vi "CMN_processOneExt.vi"(8 "error in (no error)":errorcluster, 9 "starting line":u16, 10 "str in":string) -> (0 "error out":errorcluster, 2 "number of keywords found":i32, 3 "HdrInfo":string[][](table))   [LabVIEW 2016]
doc: "This VI reads the configuration file searching for the \"infofile\" keyword. Then, it goes and reads the specified file, which should be a template for the TCS info format"
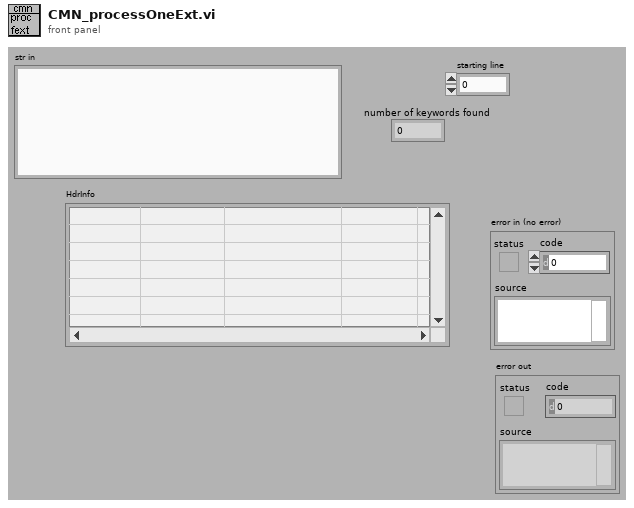
[diagram p1: front panel]
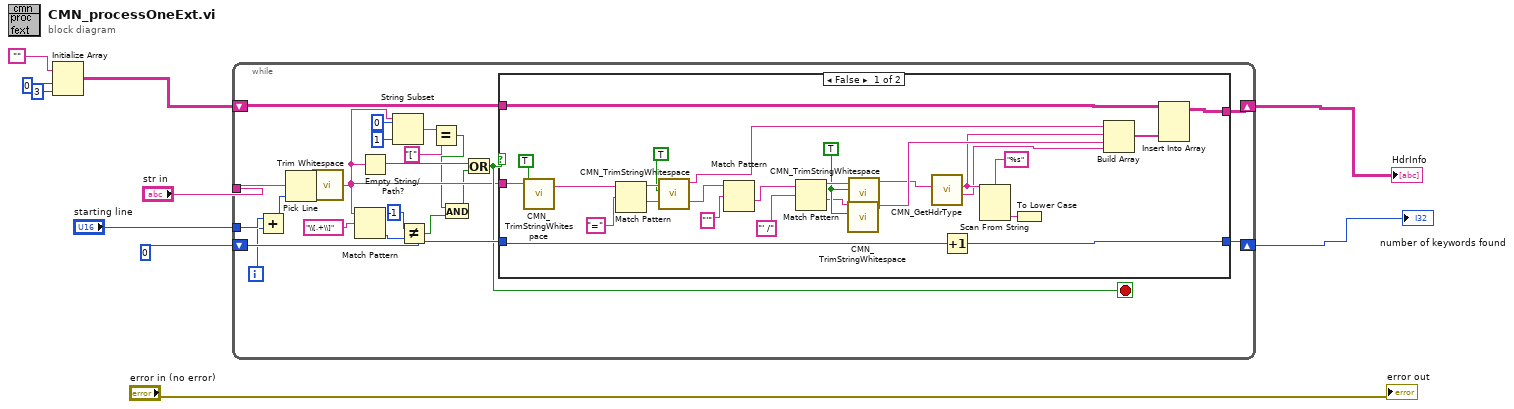
[diagram p0: block diagram]
diagram:
  n1 = Initialize Array("", 0, 3 ("dimension size")) -> (w6:string[][])
  n2 = while {
    shift-left: 0 -> [w25]
    shift-right: [w26] -> w8
    shift-left: w6 -> [w31]
    shift-right: [w30] -> w9
    tunnel: "str in" -> [w32]
    tunnel: "starting line" -> [w22]
    i -> [w21]
    stop <- w19 stop-if-true
    n3 = Add(x=w22, y=w21) -> (x+y=w20:i32)
    n4 = Pick Line(multi-line string=w32, line index=w20) -> (output string=w23:string)  [unwired: 1 out]
    n5 = call <vilib>:"Trim Whitespace.vi"("string"=w23) -> ("trimmed string"=w16:string)  [unwired: 1 in]
    n6 = Match Pattern(string=w16, regular expression="\\[.+\\]") -> (offset past match=w28:i32)  [unwired: 4 out]
    n7 = Empty String/Path?(string/path=w16) -> (empty?=w24:bool)
    n8 = String Subset(string=w16, offset (0)=0, length (rest)=1 ("length (rest)")) -> (substring=w15:string)
    n9 = Not Equal?(x=-1, y=w28) -> (x != y?=w13:bool)
    n10 = Equal?(x=w15, y="[") -> (x = y?=w12:bool)
    n11 = And(x=w12, y=w13) -> (x .and. y?=w11:bool)
    n12 = Or(x=w24, y=w11) -> (x .or. y?=w19:bool)
    n13 = case shown="False" w19 {
      tunnel: w25 -> [w42 w58]
      tunnel: w31 -> [w46 w59]
      tunnel: [w45 w59] -> w30
      tunnel: [w41 w58] -> w26
      tunnel: w16 -> [w40 _]
      frame False {
        w49 = TRUE ("Both Ends?(F)")
        n14 = call "CMN_TrimStringWhitespace.vi"("Both Ends?(T)"=TRUE ("Both Ends?(F)"), "string"=w40) -> ("trimmed string"=w39:string)  [unwired: 8 out]
        n15 = Match Pattern(string=w39, regular expression="=") -> (before substring=w56:string, after substring=w55:string)  [unwired: 3 out]
        n16 = call "CMN_TrimStringWhitespace.vi"("Both Ends?(T)"=TRUE ("Both Ends?(F)"), "string"=w56) -> ("trimmed string"=w43:string)  [unwired: 8 out]
        n17 = Match Pattern(string=w55, regular expression="'") -> (after substring=w53:string)  [unwired: 4 out]
        n18 = Match Pattern(string=w53, regular expression="' /") -> (before substring=w51:string, after substring=w48:string)  [unwired: 3 out]
        n19 = call "CMN_TrimStringWhitespace.vi"("Both Ends?(T)"=w49, "string"=w48) -> ("trimmed string"=w36:string)  [unwired: 8 out]
        n20 = call "CMN_TrimStringWhitespace.vi"("Both Ends?(T)"=w49, "string"=w51) -> ("trimmed string"=w35:string)  [unwired: 8 out]
        n21 = call "CMN_GetHdrType.vi"("keyval"=w35) -> ("type"=w33:string, "keyval out"=w34:string)  [unwired: 9 out]
        n22 = Increment(x=w42) -> (x+1=w41:i32)
        n23 = Scan From String(format string="%s", input string=w34) -> (output 1=w37:string)  [unwired: 2 in, 4 out]
        n24 = To Lower Case(string=w37) -> ()  [unwired: 1 out]
        n25 = Build Array(w43, w34, w36, w33) -> (w47:string[])
        n26 = Insert Into Array(array=w46, new element=w47) -> (w45:string[][])  [unwired: 2 in]
      }
      frame True {
      }
    }
  }
  "number of keywords found" <- w8
  "HdrInfo" <- w9
  "error out" <- "error in (no error)"
